vi "Get Type.vi"(11 "U32 1D in":refnum<class "U32 1D.lvclass">) -> (3 "Type":string)   [LabVIEW 2020, in "U32 1D.lvclass"]
uses:
  <vilib>/gpm_packages/@cs/data-type-serializer/source/U32 1D/U32 1D.lvclass
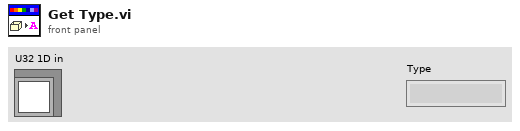
[diagram p1: front panel]
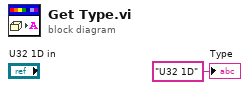
[diagram p0: block diagram]
diagram:
  "Type" <- "U32 1D" ("Type")
